vi "Test.vi"   [LabVIEW 2015, in "LibSDL2_TTF.lvlib"]
uses:
  LibSDL2_TTF.lvlib
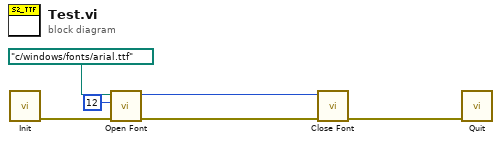
[diagram p0: block diagram]
diagram:
  n1 = call "Init.vi"() -> ("error out"=w6:errorcluster)  [unwired: 10 in, 1 out]
  n2 = call "Open Font.vi"("error in (no error)"=w6, "Size"=12, "File"=path "c:/windows/fonts/arial.ttf") -> ("error out"=w5:errorcluster, "Font Pointer"=w4:u32)  [unwired: 7 in]
  n3 = call "Close Font.vi"("error in (no error)"=w5, "Font Pointer"=w4) -> ("error out"=w3:errorcluster)  [unwired: 9 in]
  n4 = call "Quit.vi"("error in (no error)"=w3) -> ()  [unwired: 10 in, 1 out]
